vi "New.vi"(8 "Error In":errorcluster, 11 "Key":string) -> (0 "Error Out":errorcluster, 3 "Inverted Section":refnum<class "InvertedSection.lvclass">)   [LabVIEW 2018, in "Mustache.lvlib" / "Tokens.lvlib" / "InvertedSection.lvclass"]
uses:
  InvertedSection.lvclass
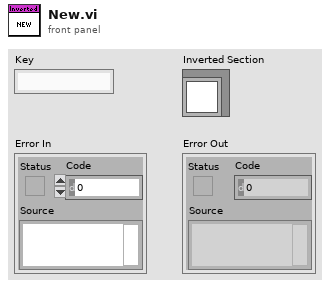
[diagram p1: front panel]
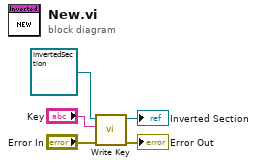
[diagram p0: block diagram]
diagram:
  n1 = call-dynamic "Write Key.vi"("Error In"="Error In", "Key"="Key", "Variable In"=refnum<class "InvertedSection.lvclass"> refnum ("Mustache.lvlib:Tokens.lvlib:InvertedSection.lvclass")) -> ("Error Out"=→"Error Out":errorcluster, "Variable Out"=→"Inverted Section":refnum<class "InvertedSection.lvclass">)  [unwired: 7 in]
